vi "Calculate Imaging Frame Rate.vi"(8 "error in (no error)":errorcluster, 10 "Frame Duration":i64=2, 11 "Durations IN":dbl[](array[numeric])) -> (0 "error out":errorcluster, 2 "LSM Frame Rate":dbl=500.0, 3 "Durations OUT":dbl[](array[numeric])=[500.0, 250.0, 500.0, 500.0, 500.0, 333.3333333333333, 500.0, 500.0, 1000.0, 500.0, 500.0, 500.0, 500.0, 500.0, 500.0, 500.0, 500.0, 500.0, 500.0, 500.0, 500.0, 500.0, 500.0, 500.0, 500.0, 500.0, 333.3333333333333, 500.0, 500.0, 500.0, 500.0, 500.0, 500.0, 500.0, 500.0, 500.0, 500.0, 500.0, 500.0, 500.0, 500.0, 500.0, 500.0, 500.0, 500.0, 1000.0, 1000.0, 500.0, 1000.0, 1000.0, 1000.0, 1000.0, 1000.0, 1000.0, 1000.0, 1000.0, 1000.0, 1000.0, 1000.0, 1000.0, 1000.0, 1000.0, 1000.0, 1000.0, 500.0, 1000.0, 500.0, 500.0, 333.3333333333333, 500.0, 500.0, 500.0, 500.0, 1000.0, 500.0, 500.0, 3.7037037037037033])   [LabVIEW 2020]
uses:
  <vilib>/Analysis/baseanly.llb/Mean (DBL).vi
  <vilib>/Analysis/NI_AALBase.lvlib
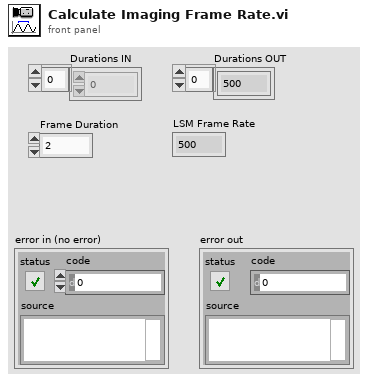
[diagram p1: front panel]
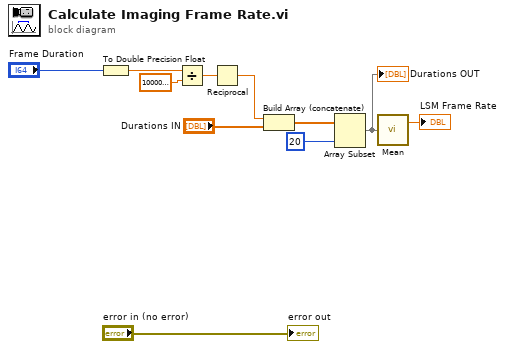
[diagram p0: block diagram]
diagram:
  n1 = To Double Precision Float(number="Frame Duration") -> (double precision float=w5:dbl)
  n2 = Divide(x=w5, y=1000000.0) -> (x/y=w6:dbl)
  n3 = Reciprocal(x=w6) -> (1/x=w2:dbl)
  n4 = Build Array (concatenate)(w2, "Durations IN") -> (w11:dbl[])
  n5 = Array Subset(array=w11, length=20) -> (w9:dbl[])  [unwired: 1 in]
  "Durations OUT" <- w9
  n6 = call-poly <vilib>:"Mean.vi"("X"=w9) -> ("mean"=→"LSM Frame Rate":dbl)  [unwired: 1 out]
  "error out" <- "error in (no error)"
